vi "TRACK.vi"(8 "error in (no error)":errorcluster, 10 "Tracking":T1, 11 "refnum in":T2) -> (0 "error out":errorcluster, 3 "refnum out":T2, 4 "question out":string)   [LabVIEW 2021, in "Korad KA3305P.lvlib"]
uses:
  Korad KA3305P.lvlib
  Reference.ctl
  Tracking.ctl
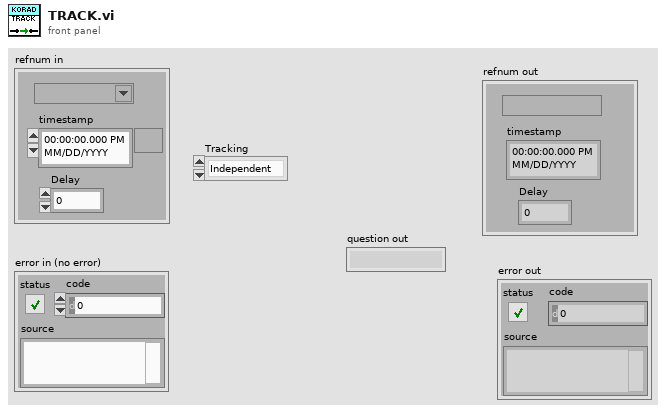
[diagram p1: front panel]
types:
  T1 = typedef "Korad KA3305P.lvlib/Tracking.ctl" = enum16{"Independent", "Serial", "Parallel"}
  T2 = typedef "Korad KA3305P.lvlib/Reference.ctl" = cluster{"refnum":refnum<visa-resource-name>, "timestamp":timestamp, "Delay":dbl}
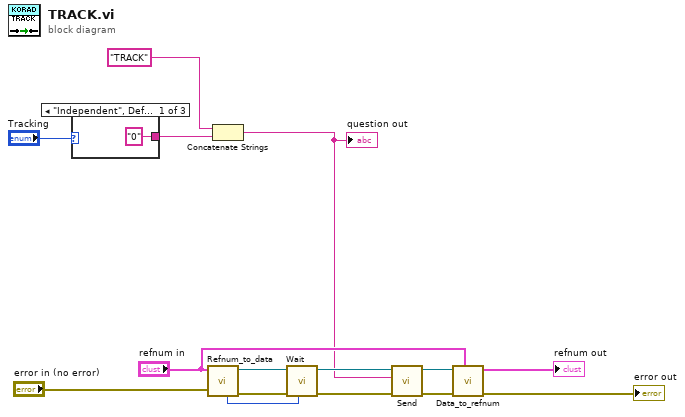
[diagram p0: block diagram]
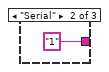
[diagram p2: hidden frame]
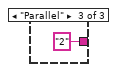
[diagram p3: hidden frame]
diagram:
  n1 = case shown="\"Independent\", Default" "Tracking" {
    tunnel: ["0" ("string") "1" ("string") "2" ("string")] -> w1
    frame "Independent", Default {
    }
    frame "Serial" {
    }
    frame "Parallel" {
    }
  }
  n2 = call "Refnum_to_data.vi"("error in (no error)"="error in (no error)", "refnum in"="refnum in") -> ("error out"=w9:errorcluster, "DAQ refnum out"=w10:refnum<visa-resource-name>, "delay out"=w11:u32)  [unwired: 7 in]
  n3 = Concatenate Strings("TRACK" ("string"), w1) -> (w4:string)
  "question out" <- w4
  n4 = call "Wait.vi"("milliseconds to wait"=w11, "error in (no error)"=w9, "refnum in"=w10) -> ("error out"=w5:errorcluster, "refnum out"=w7:refnum<visa-resource-name>)  [unwired: 7 in]
  n5 = call "Send.vi"("error in (no error)"=w5, "data"=w4, "refnum in"=w7) -> ("error out"=w8:errorcluster, "refnum out"=w13:refnum<visa-resource-name>)  [unwired: 7 in]
  n6 = call "Data_to_refnum.vi"("refnum in"="refnum in", "error in (no error)"=w8, "DAQ refnum in"=w13) -> ("error out"=→"error out":errorcluster, "refnum out"=→"refnum out":T2)  [unwired: 7 in]
